vi "VHDI-recieveCalibrationStatus.vi"(8 "error in (no error)":errorcluster, 10 "Calibration Status":T1={"Calib Status"={"Short"=FALSE, "Open"=FALSE, "Load"=FALSE, "Through"=FALSE}, "Calibrated?"=FALSE, "Permativity?"=FALSE, "Progress"={"Progress"=FALSE, "current"=enum."Short", "samples to get"=0}}, 11 "VG-VNA_GUI in":refnum<class "VG-VNA_GUI.lvclass">) -> (0 "error out":errorcluster, 3 "VG-VNA_GUI out":refnum<class "VG-VNA_GUI.lvclass">)   [LabVIEW 2020, in "VG-VNA_GUI.lvlib" / "VG-VNA_GUI.lvclass"]
uses:
  VG-VNA_GUI.lvclass
  data_handler/VDH-VNA_data_handler/VDH-VNA_data_handler/VDH-calibration_status.ctl
  data_handler/VDH-VNA_data_handler/VDH-VNA_data_handler/VDH-SOLT_calib_Status.ctl
  data_handler/VDH-VNA_data_handler/VDH-VNA_data_handler/VDH-Calibration_prosess.ctl
  data_handler/VDH-VNA_data_handler/VDH-VNA_data_handler/VDH-Calibration_enum.ctl
  data_handler/VDH-VNA_data_handler/VDH-VNA_data_handler/VDH-VNA_data_handler.lvclass
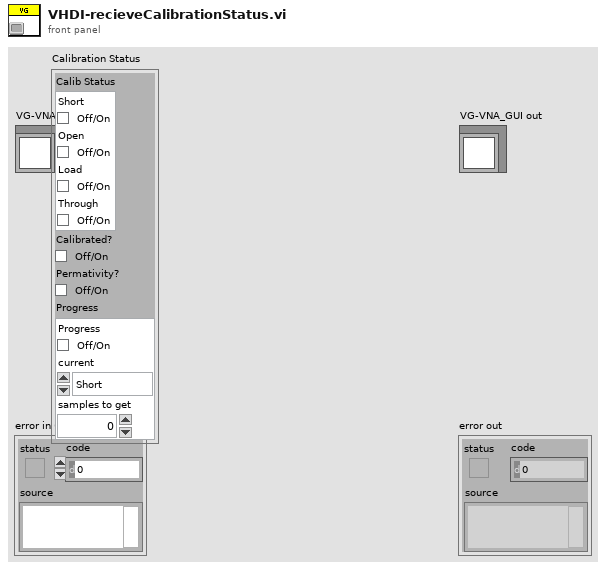
[diagram p1: front panel]
types:
  T1 = typedef "VDH-VNA_data_handler.lvlib/VDH-VNA_data_handler.lvclass/VDH-calibration_status.ctl" = cluster{"Calib Status":T2, "Calibrated?":bool, "Permativity?":bool, "Progress":T3}
  T2 = typedef "VDH-VNA_data_handler.lvlib/VDH-VNA_data_handler.lvclass/VDH-SOLT_calib_Status.ctl" = cluster{"Short":bool, "Open":bool, "Load":bool, "Through":bool}
  T3 = typedef "VDH-VNA_data_handler.lvlib/VDH-VNA_data_handler.lvclass/VDH-Calibration_prosess.ctl" = cluster{"Progress":bool, "current":T4, "samples to get":u8}
  T4 = typedef "VDH-VNA_data_handler.lvlib/VDH-VNA_data_handler.lvclass/VDH-Calibration_enum.ctl" = enum16{"Non", "Short", "Open", "Load", "Through", "Permativity"}
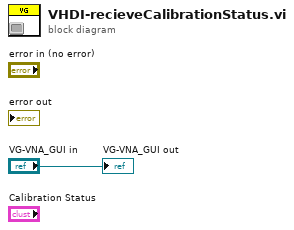
[diagram p0: block diagram]
diagram:
  "VG-VNA_GUI out" <- "VG-VNA_GUI in"
